vi "Process.vi"(8 "error in (no error)":errorcluster, 10 "Pound in":refnum<class "Pound.lvclass">, 11 "Qbus in":refnum<class "Qbus.lvclass">) -> (0 "error out":errorcluster)   [LabVIEW 2017, in "McsaDataEventCreator.lvlib"]
doc: "Creates data events and transfers data sets and trends to NI InsightCM Server."
uses:
  <vilib>/addons/InsightCM/Devices/Shared/Mcsa/McsaDataEventCreator/McsaDataEventCreator.lvlib
  <vilib>/addons/Qbus/Qbus.lvclass
  <vilib>/NI/Software Watchdog/Pound/Pound.lvclass
  <vilib>/addons/InsightCM/Devices/Shared/Mcsa/McsaDataEventCreator/controls/config.ctl
  <vilib>/addons/TimerProcess/controls/taskType.ctl
  <vilib>/NI/Software Watchdog/Watchdog/Watchdog.lvclass
  <vilib>/addons/InsightCM/Devices/Shared/Common/DataFlow/DataFlow.lvlib
  <vilib>/addons/InsightCM/Devices/Shared/Common/DataAccumulator/DataAccumulator.lvlib
  <vilib>/addons/InsightCM/Devices/Shared/Common/DataEventCreator/DataEventCreator.lvlib
  <vilib>/addons/TraceLogger/TraceLogger.lvlib
  <vilib>/addons/TimerProcess/TimerProcess.lvlib
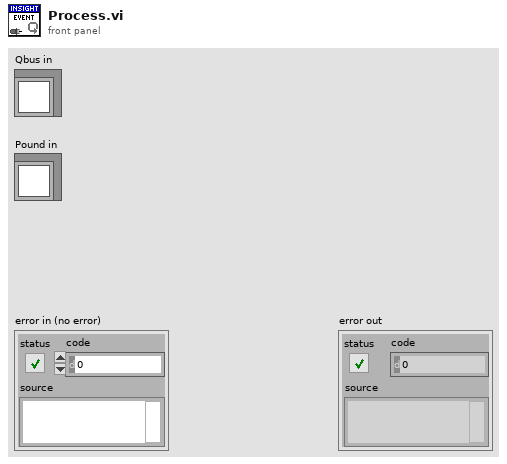
[diagram p1: front panel]
types:
  T1 = typedef "McsaDataEventCreator.lvlib/config.ctl" = cluster{"DeviceName":string, "OpenDataEvents":variant, "OpenDataEventConfigs":variant, "AcqParams":variant, "StreamIds":variant, "Registry":variant, "MaxOpenFiles":i32, "Ok To Send Data":bool}
  T2 = typedef "TimerProcess.lvlib/taskType.ctl" = enum16{"single", "repeat"}
  T3 = typedef "McsaDataEventCreator.lvlib/RegisterDataSets.ctl" = cluster{"DataGroup":string, "DataSets":T4[]}
  T4 = typedef "McsaDataEventCreator.lvlib/Registry_DataSet.ctl" = cluster{"ChannelName":string, "DataSetType":T5, "DoNotWriteToDB":bool, "ParentName":string}
  T5 = typedef "McsaDataEventCreator.lvlib/DataSetType.ctl" = enum16{"Waveform", "MCSAFFT", "TorqueWFM"}
  T6 = typedef "DataEventCreator.lvlib/RegisterTrendPoints.ctl" = cluster{"DataGroup":string, "Trends":T7[]}
  T7 = typedef "DataEventCreator.lvlib/Registry_Trend.ctl" = cluster{"TrendPointId":string, "DataSetName":string, "HighRate":bool, "Always Send":bool}
  T8 = typedef "DataFlow.lvlib/Data.ctl" = cluster{"DataGroup":string, "Waveforms":T9, "Map":T10, "Type":T11}
  T9 = typedef "wfmSGL_DVR.ctl" = refnum<data-value>
  T10 = typedef "PointValueMap.lvlib/PointMap.ctl" = refnum<data-value>
  T11 = typedef "DataFlow.lvlib/Type.ctl" = enum16{"High Rate", "Low Rate", "Burst Mode"}
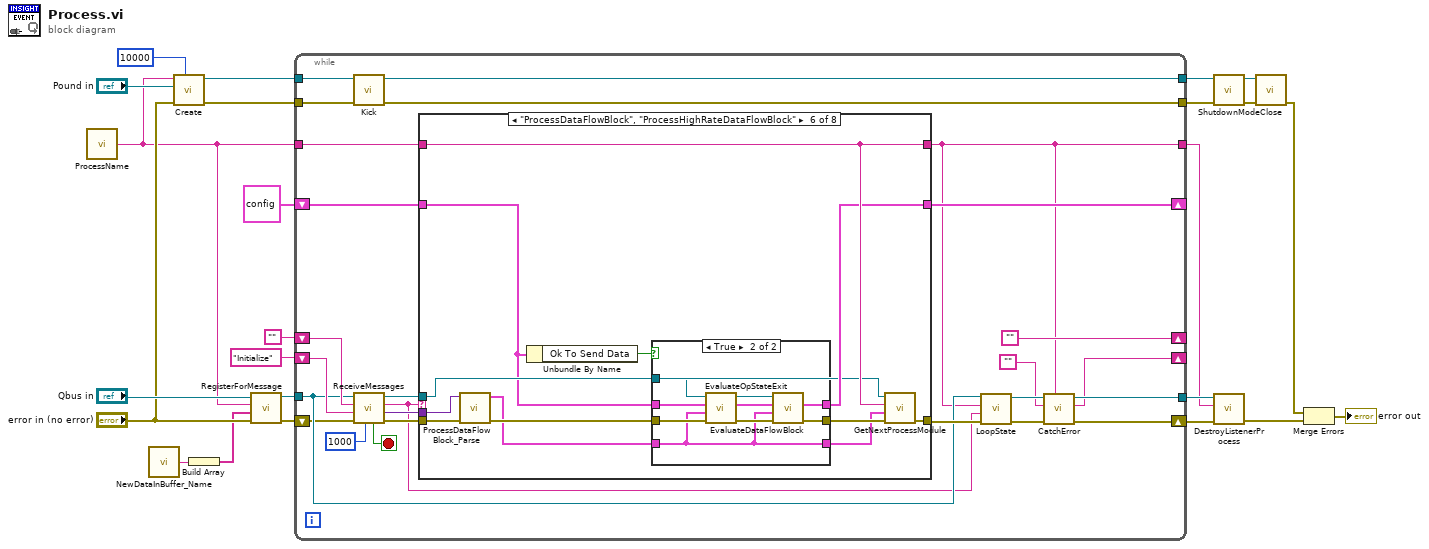
[diagram p0: block diagram]
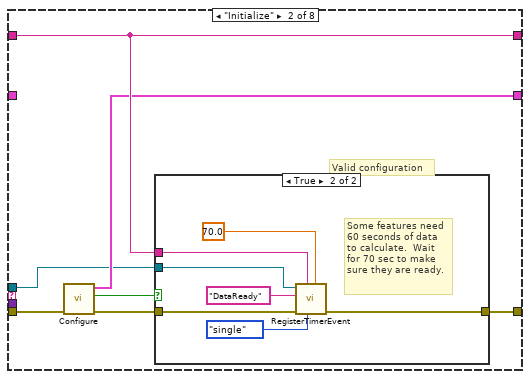
[diagram p3: hidden frame]
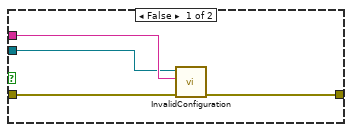
[diagram p4: hidden frame]
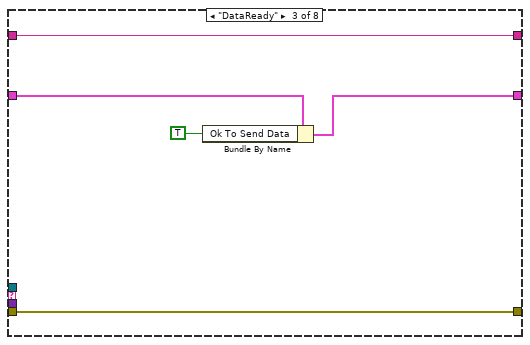
[diagram p5: hidden frame]
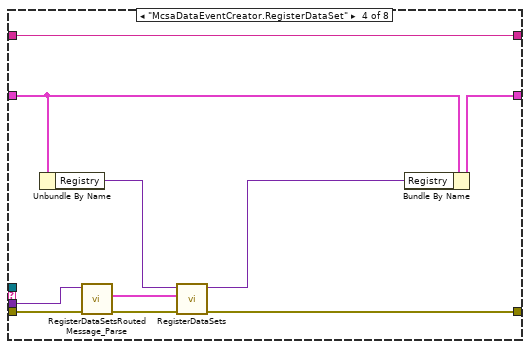
[diagram p6: hidden frame]
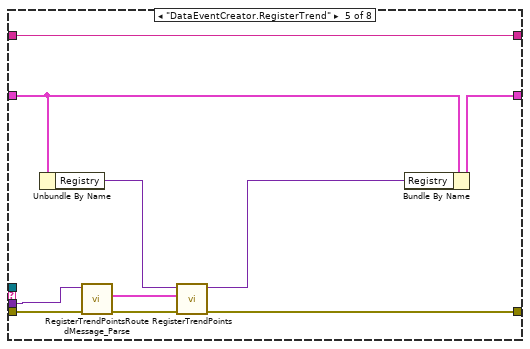
[diagram p7: hidden frame]
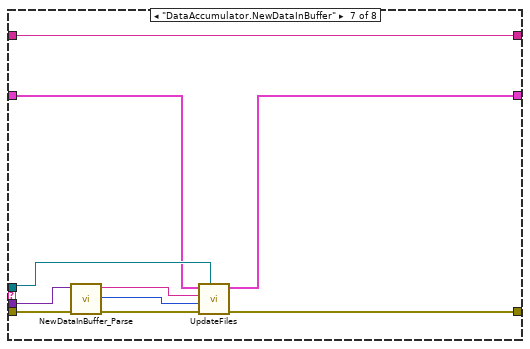
[diagram p9: hidden frame]
diagram:
  n1 = call <vilib>:"ProcessName.vi"() -> ("process name"=w1:string)  [unwired: 5 in]
  n2 = call <vilib>:"NewDataInBuffer_Name.vi"() -> ("MessageName"=w3:string)  [unwired: 5 in]
  n3 = call <vilib>:"Create.vi"("Execution Timeout (ms)"=u32 10000, "error in (no error)"="error in (no error)", "Pound"="Pound in", "Name"=w1) -> ("error out"=w9:errorcluster, "Watchdog"=w15:refnum<data-value>)  [unwired: 6 in]
  n4 = Build Array(w3) -> (w2:string[])
  n5 = call <vilib>:"RegisterForMessage.vi"("error in (no error)"="error in (no error)", "message names"=w2, "process name"=w1, "Qbus in"="Qbus in") -> ("error in (no error)"=w23:errorcluster, "Qbus out"=w22:refnum<class "Qbus.lvclass">)  [unwired: 6 in]
  n6 = while {
    shift-right: [""] -> _
    shift-left: "" -> [w49]
    tunnel: w22 -> [w37]
    tunnel: w1 -> [w27]
    tunnel: [w40] -> w20
    tunnel: [w26] -> w19
    shift-right: [w39] -> _
    shift-left: "Initialize" -> [w44]
    shift-right: [w42] -> _
    shift-left: T1 {"DeviceName"="", "OpenDataEvents"=variant(string ""), "OpenDataEventConfigs"=variant, "AcqParams"=variant, "StreamIds"=variant, "Registry"=variant, "MaxOpenFiles"=0, "Ok To Send Data"=FALSE} ("config") -> [w43]
    tunnel: w15 -> [w36]
    tunnel: [w35] -> w11
    tunnel: w9 -> [w34]
    tunnel: [w32] -> w8
    shift-right: [w41] -> w21
    shift-left: w23 -> [w33]
    stop <- w50 stop-if-true
    n7 = call <vilib>:"Kick.vi"("error in (no error)"=w34, "Watchdog"=w36) -> ("error out"=w32:errorcluster, "Watchdog"=w35:refnum<data-value>)  [unwired: 8 in]
    n8 = call <vilib>:"ReceiveMessages.vi"("Timeout(1000)"=1000 ("milliseconds to wait"), "error in (no error)"=w33, "priority action"=w44, "default action"=w49, "Qbus in"=w37) -> ("error out"=w48:errorcluster, "message value"=w45:variant, "action"=w31:string, "Qbus out"=w46:refnum<class "Qbus.lvclass">, "exit"=w50:bool)  [unwired: 2 in]
    n9 = case shown="\"ProcessDataFlowBlock\", \"ProcessHighRateDataFlowBlock\"" w31 {
      tunnel: w48 -> [w51 w60 w76 w85 w95 w107 w129 w133]
      tunnel: w46 -> [_ w54 _ _ _ w101 w124 _]
      tunnel: [w51 w58 w76 w77 w88 w106 w126 w133] -> w38
      tunnel: w45 -> [_ _ _ w84 w94 w108 w128 _]
      tunnel: w43 -> [w53 _ w75 w79 w90 w99 w122 w132]
      tunnel: [w53 w55 w74 w78 w89 w103 w123 w132] -> w42
      tunnel: [w52 w56 w72 w86 w96 w105 w130 w131] -> w26
      tunnel: w27 -> [w52 w56 w72 w86 w96 w105 w130 w131]
      frame "", Default {
      }
      frame "Initialize" {
        n10 = call <vilib>:"Configure.vi"("error in (no error)"=w60) -> ("error out"=w59:errorcluster, "valid configuration"=w57:bool, "config"=w55:T1)  [unwired: 8 in]
        n11 = case shown="True" w57 {
          tunnel: w59 -> [w61 w70]
          tunnel: [w64 w69] -> w58
          tunnel: w54 -> [w62 w71]
          tunnel: w56 -> [w63 w68]
          frame False {
            n12 = call <vilib>:"InvalidConfiguration.vi"("error in (no error)"=w61, "description"=w63, "Qbus in"=w62) -> ("error out"=w64:errorcluster)  [unwired: 7 in, 1 out]
          }
          frame True {
            # "Some features need\n60 seconds of data\nto calculate.  Wait\nfor 70 sec to make\nsure they are ready."
            # "Valid configuration"
            n13 = call <vilib>:"RegisterTimerEvent.vi"("interval (sec)"=70.0, "type"=taskType."single", "process name"=w68, "error in (no error)"=w70, "callback action"="DataReady", "qbus in"=w71) -> ("error out"=w69:errorcluster)  [unwired: 4 in, 1 out]
          }
        }
      }
      frame "DataReady" {
        n14 = Bundle By Name(cluster=w75, "Ok To Send Data"=TRUE) -> (w74:T1)
      }
      frame "McsaDataEventCreator.RegisterDataSet" {
        n15 = Unbundle By Name(w79) -> ("Registry"=w83:variant)
        n16 = call <vilib>:"RegisterDataSetsRoutedMessage_Parse.vi"("error in (no error)"=w85, "message"=w84) -> ("error out"=w81:errorcluster, "RegisterDataSet"=w82:T3)  [unwired: 8 in]
        n17 = call <vilib>:"RegisterDataSets.vi"("error in (no error)"=w81, "RegisterDataSet"=w82, "registry in"=w83) -> ("error out"=w77:errorcluster, "registry out"=w80:variant)  [unwired: 7 in]
        n18 = Bundle By Name(cluster=w79, "Registry"=w80) -> (w78:T1)
      }
      frame "DataEventCreator.RegisterTrend" {
        n19 = Unbundle By Name(w90) -> ("Registry"=w93:variant)
        n20 = call <vilib>:"RegisterTrendPointsRoutedMessage_Parse.vi"("error in (no error)"=w95, "message"=w94) -> ("error out"=w92:errorcluster, "RegisterTrend"=w87:T6)  [unwired: 8 in]
        n21 = call <vilib>:"RegisterTrendPoints.vi"("error in (no error)"=w92, "register trend"=w87, "registry in"=w93) -> ("error out"=w88:errorcluster, "registry out"=w91:variant)  [unwired: 7 in]
        n22 = Bundle By Name(cluster=w90, "Registry"=w91) -> (w89:T1)
      }
      frame "ProcessDataFlowBlock", "ProcessHighRateDataFlowBlock" {
        n23 = call <vilib>:"ProcessDataFlowBlock_Parse.vi"("error in (no error)"=w107, "body"=w108) -> ("error out"=w102:errorcluster, "data"=w100:T8)  [unwired: 8 in]
        n24 = Unbundle By Name(w99) -> ("Ok To Send Data"=w97:bool)
        n25 = case shown="True" w97 {
          tunnel: [w111 w120] -> w104
          tunnel: [w110 w119] -> w103
          tunnel: w99 -> [w110 w118]
          tunnel: w102 -> [w111 w117]
          tunnel: w101 -> [_ w116]
          tunnel: w100 -> [w109 w112]
          tunnel: [w109 w112] -> w98
          frame False {
          }
          frame True {
            n26 = call <vilib>:"EvaluateOpStateExit.vi"("error in (no error)"=w117, "data"=w112, "config in"=w118, "Qbus in"=w116) -> ("error out"=w115:errorcluster, "config out"=w113:T1, "Qbus out"=w114:refnum<class "Qbus.lvclass">)  [unwired: 5 in]
            n27 = call <vilib>:"EvaluateDataFlowBlock.vi"("error in (no error)"=w115, "data"=w112, "config"=w113, "Qbus"=w114) -> ("error out"=w120:errorcluster, "config"=w119:T1)  [unwired: 6 in]
          }
        }
        n28 = call <vilib>:"GetNextProcessModule.vi"("error in (no error)"=w104, "data"=w98, "source"=w105, "Qbus in"=w101) -> ("error out"=w106:errorcluster)  [unwired: 6 in, 1 out]
      }
      frame "DataAccumulator.NewDataInBuffer" {
        n29 = call <vilib>:"NewDataInBuffer_Parse.vi"("error in (no error)"=w129, "Message"=w128) -> ("error out"=w127:errorcluster, "buffer location"=w125:u32, "data group"=w121:string)  [unwired: 7 in]
        n30 = call <vilib>:"UpdateFiles.vi"("Qbus"=w124, "error in (no error)"=w127, "buffer location"=w125, "data group"=w121, "config"=w122) -> ("error out"=w126:errorcluster, "config"=w123:T1)  [unwired: 5 in]
      }
      frame "Exit" {
      }
    }
    n31 = call <vilib>:"LoopState.vi"("error in (no error)"=w38, "loop action"=w31, "process name"=w26, "Qbus in"=w37) -> ("error out"=w29:errorcluster, "Qbus out"=w28:refnum<class "Qbus.lvclass">)  [unwired: 6 in]
    n32 = call <vilib>:"CatchError.vi"("source"=w26, "error in (no error)"=w29, "next action in"="", "Qbus in"=w28) -> ("error out"=w41:errorcluster, "next action out"=w39:string, "Qbus out"=w40:refnum<class "Qbus.lvclass">)  [unwired: 5 in]
  }
  n33 = call <vilib>:"ShutdownMode.vi"("error in (no error)"=w8, "Watchdog"=w11) -> ("error out"=w10:errorcluster, "Watchdog"=w12:refnum<data-value>)  [unwired: 8 in]
  n34 = call <vilib>:"DestroyListenerProcess.vi"("error in (no error)"=w21, "process name"=w19, "Qbus in"=w20) -> ("error in (no error)"=w7:errorcluster)  [unwired: 7 in, 1 out]
  n35 = call <vilib>:"Close.vi"("error in (no error)"=w10, "Watchdog"=w12) -> ("error out"=w6:errorcluster)  [unwired: 9 in]
  n36 = Merge Errors(w6, w7) -> (→"error out":errorcluster)
